vi "Filter Entity Paths.vi"(11 "Class Paths":path[](array[path])) -> (0 "error out":errorcluster, 2 "Names":string[](array[string]), 3 "Entity Paths":path[](array[path]))   [LabVIEW 2020, in "Conditum-Tools.lvlib" / "Entity Editor.lvclass"]
uses:
  Entity Editor.lvclass
  33505b48-b9bf-4e0d-8919-721f358d0b44.vi
  977a2201-4cc6-4a54-9c30-d8d2a5040881.vi
  Filter Entity Paths OoC.vi
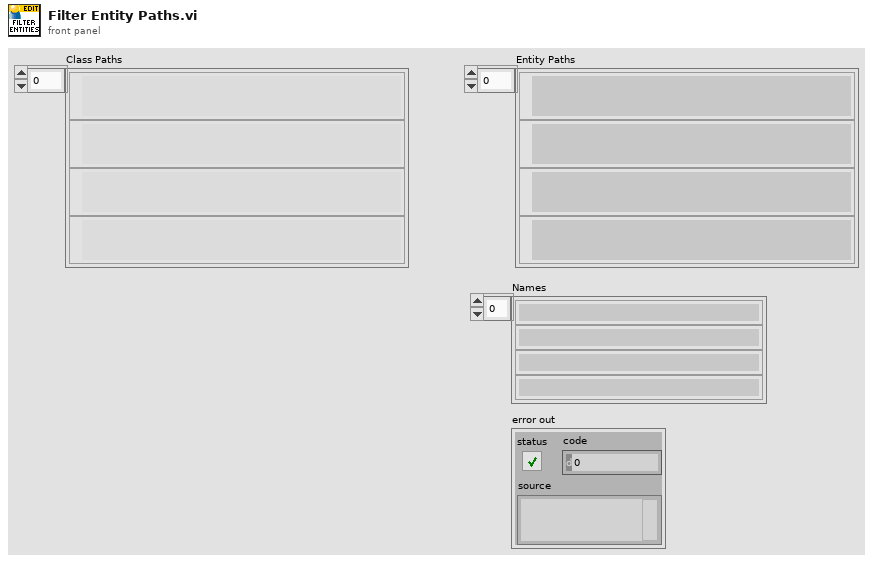
[diagram p1: front panel]
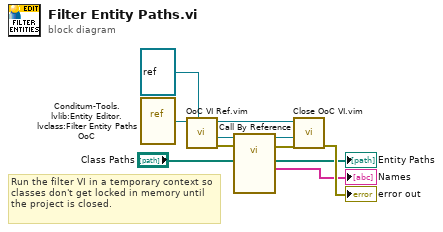
[diagram p0: block diagram]
diagram:
  # "Run the filter VI in a temporary context so classes don't get locked in memory until the project is closed."
  n1 = vi-ref "Conditum-Tools.lvlib:Entity Editor.lvclass:Filter Entity Paths OoC.vi"() -> (w6:refnum<vi>)
  n2 = call "OoC VI Ref.vim"("VI Type"=refnum<vi> refnum, "OoC SVR"=w6) -> ("error out"=w9:errorcluster, "vi reference"=w10:refnum<vi>, "context"=w8:refnum<vi>)  [unwired: 7 in]
  n3 = call-by-ref "?"(reference=w10, error in=w9, "Class Paths"="Class Paths") -> (reference out=w7:refnum<vi>, error out=w1:errorcluster, "Names"=→"Names":string[], "Entity Paths"=→"Entity Paths":path[])  [unwired: 9 in]
  n4 = call "Close OoC VI.vim"("error in (no error)"=w1, "vi reference"=w7, "context"=w8) -> ("error out"=→"error out":errorcluster)  [unwired: 8 in]
